vi "VI_CallingVI_WithXControl.vi"(11 "Numeric":dbl) -> (3 "Numeric 2":dbl)   [LabVIEW 2012]
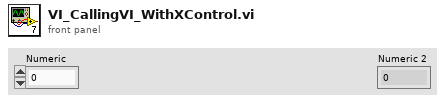
[diagram p1: front panel]
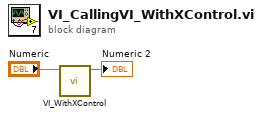
[diagram p0: block diagram]
diagram:
  n1 = call "VI_WithXControl.vi"("Min Max Slider XControl"="Numeric") -> ("Min Max Slider XControl 2"=→"Numeric 2":dbl)  [unwired: 10 in]
